vi "LEP_RV_CheckDebug.vi"(7 "Enable debugging":bool, 8 "error in (no error)":errorcluster, 11 "VI Refnum":refnum<vi>) -> (0 "error out":errorcluster, 3 "VI Refnum out":refnum<vi>)   [LabVIEW 2011]
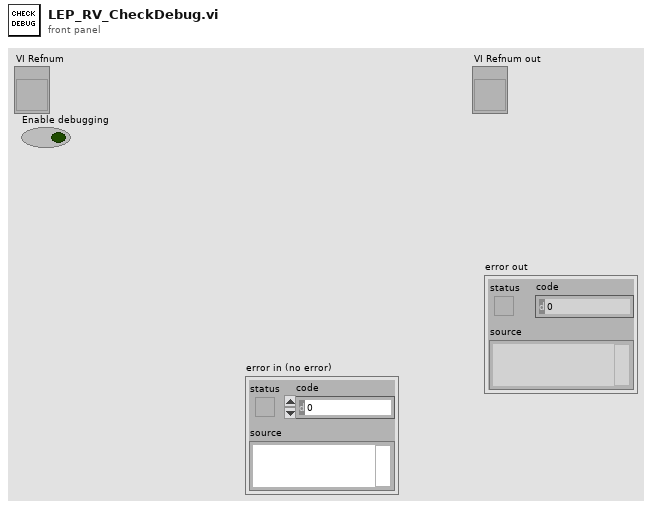
[diagram p1: front panel]
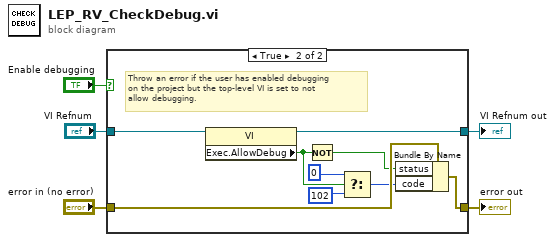
[diagram p0: block diagram]
diagram:
  n1 = case shown="True" "Enable debugging" {
    tunnel: "VI Refnum" -> [w7 w16]
    tunnel: [w7 w15] -> w3
    tunnel: "error in (no error)" -> [w6 w14]
    tunnel: [w6 w13] -> w1
    frame False {
    }
    frame True {
      # "Throw an error if the user has enabled debugging\non the project but the top-level VI is set to not\nallow debugging."
      n2 = property class="VI"(reference=w16) -> (reference out=w15:refnum<vi>, "Exec.AllowDebug"=w11:bool)  [unwired: 1 in, 1 out]
      n3 = Not(x=w11) -> (.not. x?=w12:bool)
      n4 = Select(t=0 ("code"), s=w11, f=102 ("code")) -> (s? t:f=w8:i32)
      n5 = Bundle By Name(cluster=w14, "status"=w12, "code"=w8) -> (w13:errorcluster)
    }
  }
  "VI Refnum out" <- w3
  "error out" <- w1
